vi "Init.vi"(8 "error in (no error)":errorcluster, 11 "Hotkey Name":string) -> (0 "error out":errorcluster, 3 "TriggerHotkeyByName out":refnum<class "TriggerHotkeyByName.lvclass">)   [LabVIEW 2020, in "obs-websocket.lvlib" / "TriggerHotkeyByName.lvclass"]
uses:
  TriggerHotkeyByName.lvclass
  TriggerHotkeyByName.lvclass/TriggerHotkeyByName.ctl
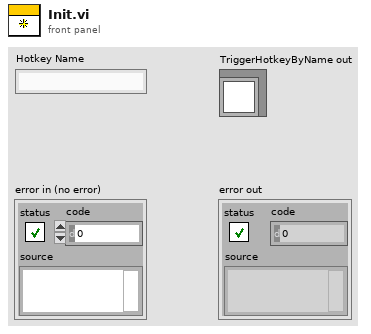
[diagram p1: front panel]
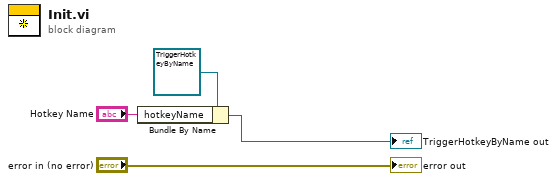
[diagram p0: block diagram]
diagram:
  n1 = Bundle By Name(cluster=refnum<class "TriggerHotkeyByName.lvclass"> refnum ("TriggerHotkeyByName in"), "hotkeyName"="Hotkey Name") -> (→"TriggerHotkeyByName out":refnum<class "TriggerHotkeyByName.lvclass">)
  "error out" <- "error in (no error)"
